vi "Variant_GetName.vi"(11 "Variant":variant) -> (1 "found":bool, 2 "Name":string, 3 "Variant dup":variant)   [LabVIEW 2013, in "OpenVariant.lvlib"]
uses:
  OpenVariant.lvlib
  <vilib>/Utility/VariantDataType/TypedefInfo.ctl
  TypeDescriptor/OpenDescriptor.lvlib
  <vilib>/Utility/VariantDataType/VariantType.lvlib
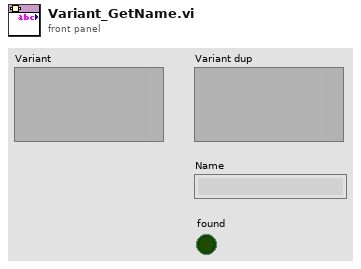
[diagram p1: front panel]
types:
  T1 = typedef "VariantType.lvlib/TypedefInfo.ctl" = cluster{"Name":string, "Timestamp":u32}
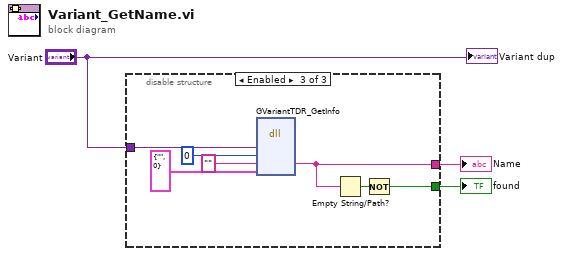
[diagram p0: block diagram]
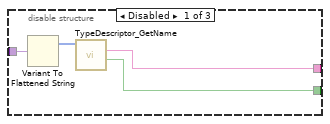
[diagram p2: hidden frame]
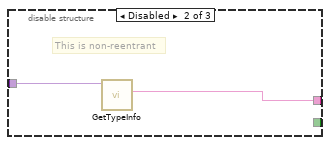
[diagram p3: hidden frame]
diagram:
  n1 = disable-structure shown="Enabled" {
    disable-tunnel: "Variant" -> [w6 w9 w12]
    disable-tunnel: [w4 _ w11] -> w2
    disable-tunnel: [w5 w8 w10] -> w1
    frame Disabled {
      n2 = Variant To Flattened String(Variant=w6) -> (1:w7:i16[])  [unwired: 1 out]
      n3 = call "TypeDescriptor_GetName.vi"("type descriptor"=w7) -> ("found"=w4:bool, "name"=w5:string)  [unwired: 8 in, 1 out]
    }
    frame Disabled {
      # "This is non-reentrant"
      n4 = call <vilib>:"GetTypeInfo.vi"("Variant"=w9) -> ("Name"=w8:string)  [unwired: 6 in, 4 out]
    }
    frame Enabled {
      n5 = dll-call lib="LabVIEW" fn="GVariantTDR_GetInfo"("lvVar"=w12, "typeCode"=i16 0, "name"="", "typeDef"=T1 {"Name"="", "Timestamp"=0} ("TypedefInfo")) -> ("name"=w10:string)  [unwired: 4 in, 5 out]
      n6 = Empty String/Path?(string/path=w10) -> (empty?=w16:bool)
      n7 = Not(x=w16) -> (.not. x?=w11:bool)
    }
  }
  "Name" <- w1
  "found" <- w2
  "Variant dup" <- "Variant"
